vi "Coord window-Clear.vi"(8 "error in (no error)":errorcluster, 11 "No dialogue":bool) -> (0 "error out":errorcluster)   [LabVIEW 2013]
uses:
  Globals/Coord window-Globals.vi
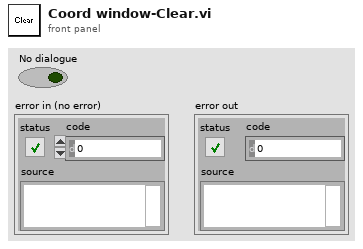
[diagram p1: front panel]
types:
  T1 = cluster{"Caption-Right button":string, "Caption-Left button":string, "Message to display":string, "Delay before close":u32, "Window Colour":u32, "Cancel button disabled?":enum8{"Enabled", "Disabled", "Disabled and Grayed Out"}}
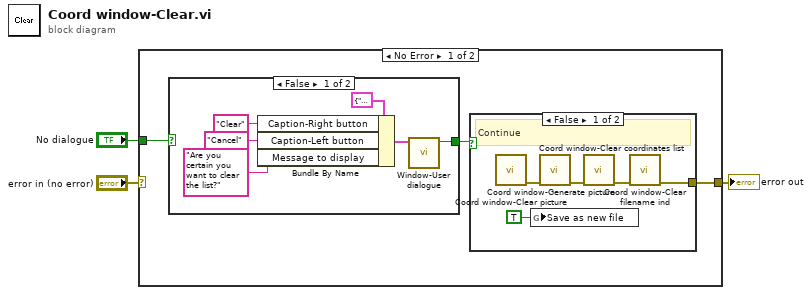
[diagram p0: block diagram]
diagram:
  n1 = case shown="No Error" "error in (no error)" {
    selector: "error in (no error)" -> [_ w18]
    tunnel: [w6 w18] -> w3
    tunnel: "No dialogue" -> [w4 _]
    frame No Error {
      n2 = case shown="False" w4 {
        tunnel: [w7 _] -> w5
        frame False {
          n3 = Bundle By Name(cluster=T1 {"Caption-Right button"="Add duplicate", "Caption-Left button"="Cancel", "Message to display"="", "Delay before close"=0, "Window Colour"=16448250, "Cancel button disabled?"=enum."Enabled"} ("Input cluster"), "Caption-Right button"="Clear", "Caption-Left button"="Cancel", "Message to display"="Are you certain you want to clear the list?") -> (w12:T1)
          n4 = call "Window-User dialogue.vi"("Input cluster"=w12) -> ("Left Button (Cancel)"=w7:bool)  [unwired: 10 in]
        }
        frame True {
        }
      }
      n5 = case shown="False" w5 {
        tunnel: [w13 _] -> w6
        frame False {
          # "Continue"
          n6 = call "Coord window-Clear picture.vi"() -> ("error out"=w16:errorcluster)  [unwired: 11 in]
          n7 = global write "Coord window-Globals.vi" "Save as new file"(TRUE ("Save as new file")) -> ()
          n8 = call "Coord window-Clear coordinates list.vi"("error in (no error)"=w16) -> ("error out"=w17:errorcluster)  [unwired: 10 in]
          n9 = call "Coord window-Generate picture.vi"("error in (no error)"=w17) -> ("error out"=w14:errorcluster)  [unwired: 10 in]
          n10 = call "Coord window-Clear filename ind.vi"("error in (no error)"=w14) -> ("error out"=w13:errorcluster)  [unwired: 10 in]
        }
        frame True {
          # "Cancelled"
        }
      }
    }
    frame Error {
    }
  }
  "error out" <- w3
